vi "Stop Processes.vi"(8 "error in (no error)":errorcluster, 9 "timeout in ms (-1)":i32=-1, 11 "Application In":refnum<class "Application.lvclass">) -> (0 "error out":errorcluster, 1 "Timed out?":bool, 3 "Application Out":refnum<class "Application.lvclass">)   [LabVIEW 2020, in "Application.lvclass"]
uses:
  Application.lvclass
  Application.lvclass/Application.ctl
  Process/Process.lvclass/Process.ctl
  Process/Public/Get Lifecycle State.vi
  Process/Private/SubVIs/Wait for finish.vi
  Process/Protected/Messaging/Enqueue Message.vi
  Process/Private/SubVIs/Set Lifecycle State.vi
  <vilib>/Utility/error.llb/Clear Errors.vi
  <vilib>/Utility/error.llb/Error Cluster From Error Code.vi
  Process/Process.lvclass
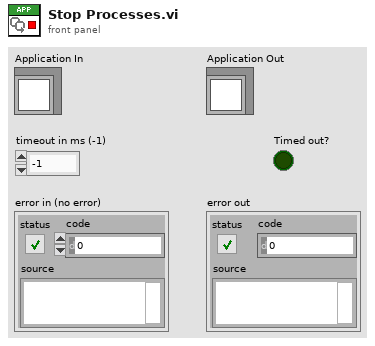
[diagram p1: front panel]
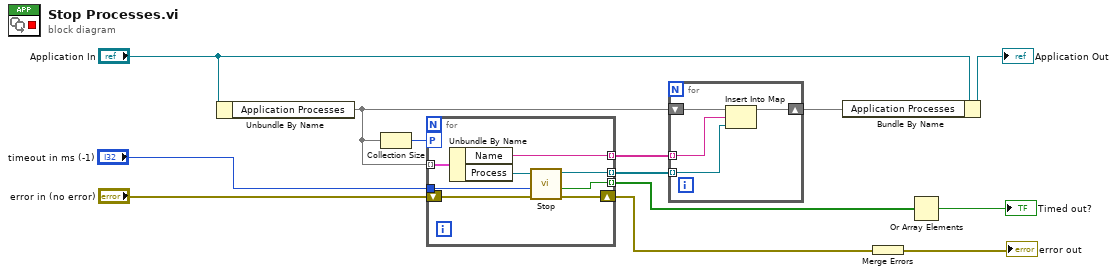
[diagram p0: block diagram]
diagram:
  n1 = Unbundle By Name("Application In") -> ("Application Processes"=w3:map{string, refnum<class "Process.lvclass">})
  n2 = Collection Size(1:w3) -> (0:w5:i32)
  n3 = for {
    tunnel: "timeout in ms (-1)" -> [w19]
    tunnel: [w18] -> w10 mode=indexing
    shift-right: [w21] -> w12
    shift-left: "error in (no error)" -> [w20]
    tunnel: w3 -> [w17] mode=indexing
    workers-P: w5 -> [_]
    tunnel: [w15] -> w2 mode=indexing
    tunnel: [w14] -> w1 mode=indexing
    n4 = Unbundle By Name(w17) -> ("Name"=w15:string, "Process"=w16:refnum<class "Process.lvclass">)
    n5 = call "Stop.vi"("error in (no error)"=w20, "timeout in ms (-1)"=w19, "Process In"=w16) -> ("error out"=w21:errorcluster, "timed out?"=w18:bool, "Process Out"=w14:refnum<class "Process.lvclass">)  [unwired: 6 in]
  }
  n6 = for {
    shift-right: [w24] -> w4
    shift-left: w3 -> [w25]
    tunnel: w2 -> [w23] mode=indexing
    tunnel: w1 -> [w22] mode=indexing
    n7 = Insert Into Map(map in=w25, key=w23, value=w22) -> (map out=w24:map{string, refnum<class "Process.lvclass">})  [unwired: 2 out]
  }
  n8 = Bundle By Name(cluster="Application In", "Application Processes"=w4) -> (→"Application Out":refnum<class "Application.lvclass">)
  n9 = Merge Errors(w12) -> (→"error out":errorcluster)
  n10 = Or Array Elements(Boolean array=w10) -> (logical OR=→"Timed out?":bool)
